vi "Format Errors.vi"(8 "error in (no error)":errorcluster[](array[cluster]), 11 "SigMan in":refnum<class "SignalManager.lvclass">) -> (0 "error out":errorcluster, 3 "SigMan out":refnum<class "SignalManager.lvclass">)   [LabVIEW 2015, in "SignalManager.lvclass"]
uses:
  SignalManager.lvclass
  SignalManager.lvclass/SignalManager.ctl
  <vilib>/regexp/Match Regular Expression.xnode
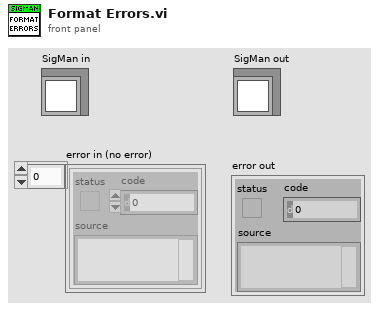
[diagram p1: front panel]
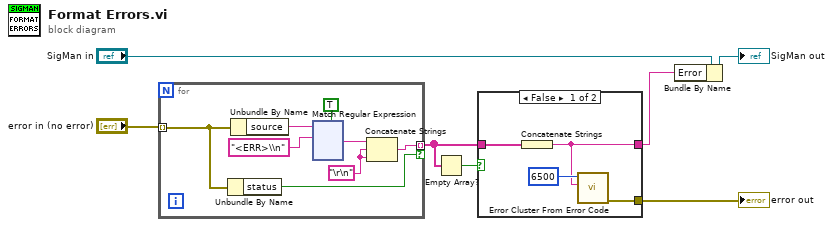
[diagram p0: block diagram]
diagram:
  n1 = for {
    tunnel: "error in (no error)" -> [w11] mode=indexing
    tunnel: [w9] -> w4 mode=indexing if=w10
    w8 = "\r\n"
    n2 = Unbundle By Name(w11) -> ("status"=w10:bool)
    n3 = Unbundle By Name(w11) -> ("source"=w14:string)
    n4 = xnode "Match Regular Expression"("input string"=w14, "regular expression"="<ERR>\\n", "multiline? (F)"=TRUE) -> ("after match"=w13:string)  [unwired: 3 in, 4 out]
    n5 = Concatenate Strings(w13, w8, w8) -> (w9:string)
  }
  n6 = Empty Array?(array=w4) -> (empty?=w3:bool)
  n7 = case shown="False" w3 {
    tunnel: [w133 _] -> w5
    tunnel: w4 -> [w132 _]
    tunnel: [w130 _] -> w1
    frame False {
      n8 = Concatenate Strings(w132) -> (w130:string)
      n9 = call <vilib>:"Error Cluster From Error Code.vi"("error message (\"\")"=w130, "error code (0)"=6500) -> ("error out"=w133:errorcluster)  [unwired: 7 in]
    }
    frame True {
    }
  }
  "error out" <- w5
  n10 = Bundle By Name(cluster="SigMan in", "Error"=w1) -> (→"SigMan out":refnum<class "SignalManager.lvclass">)
